vi "ma_extend resamp open-interval to close-interval.vi"(5 "closed interval asymmetric":bool=TRUE, 6 "t0 WDT in":timestamp, 7 "open interval? (T)":bool, 8 "error in":errorcluster, 9 "t0 user":timestamp, 10 "original waveform in":waveform(dbl)={"t0"=timestamp(0 s since 1904-01-01), "dt"=0.0, "Y"=[]}, 11 "resampled waveform in":waveform(dbl)={"t0"=timestamp(0 s since 1904-01-01), "dt"=0.0, "Y"=[]}) -> (0 "error out":errorcluster, 1 "t0 modified":timestamp, 3 "Waveform out":waveform(dbl), 4 "t0 adjusted":bool)   [LabVIEW 2020, in "NI_MAPro.lvlib"]
uses:
  NI_MAPro.lvlib
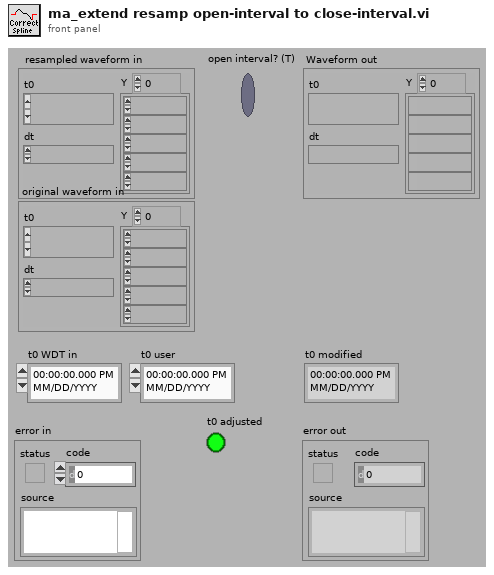
[diagram p1: front panel]
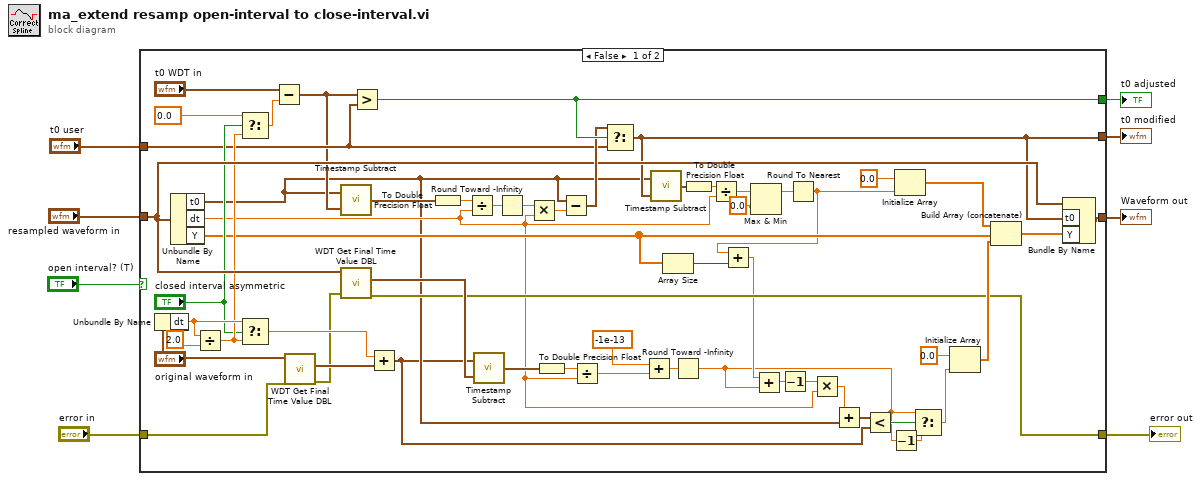
[diagram p0: block diagram]
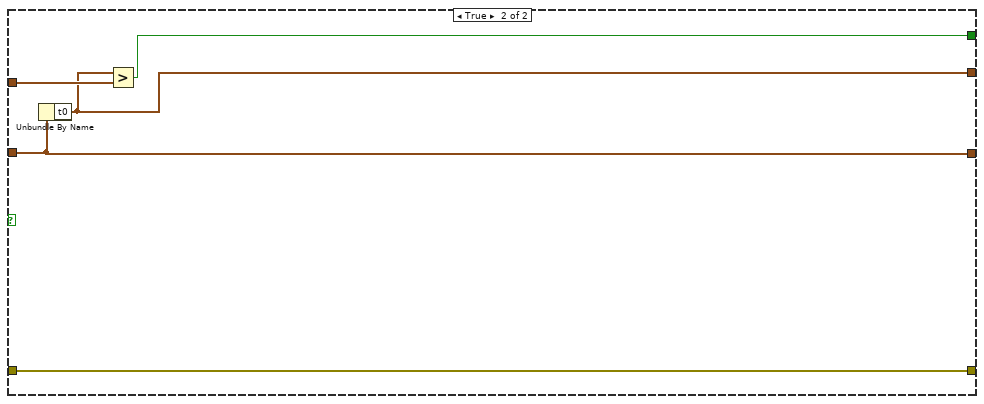
[diagram p2: hidden frame]
diagram:
  n1 = case shown="False" "open interval? (T)" {
    tunnel: [w59 w69] -> w6
    tunnel: "resampled waveform in" -> [w51 w69]
    tunnel: "t0 user" -> [w32 w68]
    tunnel: [w63 w67] -> w4
    tunnel: [w35 w66] -> w3
    tunnel: "error in" -> [w27 w65]
    tunnel: [w24 w65] -> w1
    frame False {
      n2 = Unbundle By Name("original waveform in") -> ("dt"=w41:dbl)
      n3 = Unbundle By Name(w51) -> ("t0"=w15:timestamp, "dt"=w17:dbl, "Y"=w23:dbl[])
      n4 = Divide(x=w41, y=2.0) -> (x/y=w40:dbl)
      n5 = Select(t=0.0 ("y"), s="closed interval asymmetric", f=w40) -> (s? t:f=w38:dbl)
      n6 = Select(t=w41, s="closed interval asymmetric", f=w40) -> (s? t:f=w42:dbl)
      n7 = Subtract(x="t0 WDT in", y=w38) -> (x-y=w25:timestamp)
      n8 = call "WDT Get Final Time Value DBL.vi"("error in (no error)"=w27, "waveform in"="original waveform in") -> ("error out"=w26:errorcluster, "tf"=w47:timestamp)  [unwired: 7 in, 1 out]
      n9 = call "Timestamp Subtract.vi"("y"=w25, "x"=w15) -> ("x - y"=w62:timestamp)
      n10 = call "WDT Get Final Time Value DBL.vi"("error in (no error)"=w26, "waveform in"=w51) -> ("error out"=w24:errorcluster, "tf"=w30:timestamp)  [unwired: 7 in, 1 out]
      n11 = Greater?(x=w25, y=w32) -> (0:w63:bool)
      n12 = Add(x=w42, y=w47) -> (x+y=w13:timestamp)
      n13 = To Double Precision Float(number=w62) -> (double precision float=w31:dbl)
      n14 = Divide(x=w31, y=w17) -> (x/y=w28:dbl)
      n15 = call "Timestamp Subtract.vi"("y"=w30, "x"=w13) -> ("x - y"=w33:timestamp)
      n16 = Round Toward -Infinity(1:w28) -> (0:w56:dbl)
      n17 = Multiply(x=w56, y=w17) -> (x*y=w60:dbl)
      n18 = To Double Precision Float(number=w33) -> (double precision float=w34:dbl)
      n19 = Subtract(x=w15, y=w60) -> (x-y=w57:timestamp)
      n20 = Divide(x=w34, y=w17) -> (x/y=w45:dbl)
      n21 = Select(t=w57, s=w63, f=w32) -> (s? t:f=w35:timestamp)
      n22 = Add(x=-1e-13 ("y"), y=w45) -> (x+y=w44:dbl)
      n23 = call "Timestamp Subtract.vi"("y"=w35, "x"=w15) -> ("x - y"=w55:timestamp)
      n24 = Array Size(array=w23) -> (size(s)=w22:i32)
      n25 = Round Toward -Infinity(1:w44) -> (0:w11:dbl)
      n26 = To Double Precision Float(number=w55) -> (double precision float=w29:dbl)
      n27 = Divide(x=w29, y=w17) -> (x/y=w54:dbl)
      n28 = Max & Min(x=w54, y=0.0) -> (max(x,y)=w53:dbl)  [unwired: 1 out]
      n29 = Round To Nearest(number=w53) -> (nearest integer value=w21:dbl)
      n30 = Add(x=w21, y=w22) -> (x+y=w20:dbl)
      n31 = Add(x=w20, y=w11) -> (x+y=w19:dbl)
      n32 = Decrement(x=w19) -> (x-1=w18:dbl)
      n33 = Multiply(x=w18, y=w17) -> (x*y=w16:dbl)
      n34 = Add(x=w16, y=w15) -> (x+y=w14:timestamp)
      n35 = Less?(x=w14, y=w13) -> (x < y?=w12:bool)
      n36 = Decrement(x=w11) -> (x-1=w10:dbl)
      n37 = Initialize Array(0.0 ("element"), w21) -> (w58:dbl[])
      n38 = Select(t=w11, s=w12, f=w10) -> (s? t:f=w9:dbl)
      n39 = Initialize Array(0.0 ("y"), w9) -> (w36:dbl[])
      n40 = Build Array (concatenate)(w58, w23, w36) -> (w50:dbl[])
      n41 = Bundle By Name(cluster=w51, "t0"=w35, "Y"=w50) -> (w59:waveform(dbl))
    }
    frame True {
      n42 = Unbundle By Name(w69) -> ("t0"=w66:timestamp)
      n43 = Greater?(x=w66, y=w68) -> (0:w67:bool)
    }
  }
  "Waveform out" <- w6
  "t0 modified" <- w3
  "error out" <- w1
  "t0 adjusted" <- w4
